vi "Count LEDs.vi"(8 "error in (no error)":errorcluster, 11 "LED Board Visual Test in":refnum<class "LED Board Test.lvclass">) -> (0 "error out":errorcluster, 2 "Fail Codes":string, 3 "Tests Passed":bool)   [LabVIEW 2015, in "LED Board Test.lvclass"]
uses:
  LED Board Test.lvclass
  LED Board Test.lvclass/LED Board Test.ctl
  Classes/Test Recipe/Class/Test Recipe.lvclass
  <vilib>/Cree, Inc/Cree Test Framework/Core Launcher/Core Launcher.lvlib
  <vilib>/Cree, Inc/Cree Test Framework/Classes/Data/Data Repo/Class/Data Repo.lvclass
  Classes/Application/Class/Application.lvclass
  Test Class/Test Class.lvclass
  Classes/Station Config/Class/Station Config.lvclass
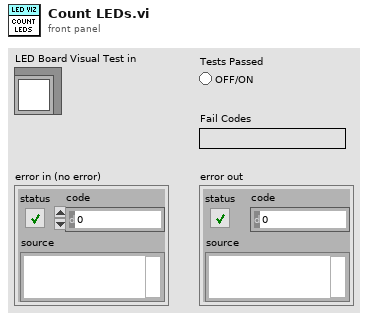
[diagram p1: front panel]
types:
  T1 = typedef "Application.lvlib/App Properties.lvclass/Class Properties -- Cluster.ctl" = cluster{"UUT Info":T2[], "Test Information":refnum<vi>, "Test Complete Event":refnum<user-event>, "Shop Floor System":refnum<class "Shop Floor System.lvclass">, "Gold Board":refnum<class "Golden Board.lvclass">, "Test Recipe":refnum<class "Test Recipe.lvclass">, "Instruments":refnum<class "Instrument.lvclass">[], "Mode":T3, "Test Results":T4[], "Station Config":refnum<class "Station Config.lvclass">}
  T2 = typedef "Application.lvlib/App Properties.lvclass/UUT Reference -- Cluster.ctl" = cluster{"Serial Number Reference":refnum<vi>, "Status Message Reference":refnum<vi>}
  T3 = typedef "Application.lvlib/Application.lvclass/Op Mode -- Enum.ctl" = u16
  T4 = typedef "Application.lvlib/App Properties.lvclass/Test Result -- Cluster.ctl" = cluster{"Position":i32, "Pass":bool, "Fail Codes":string}
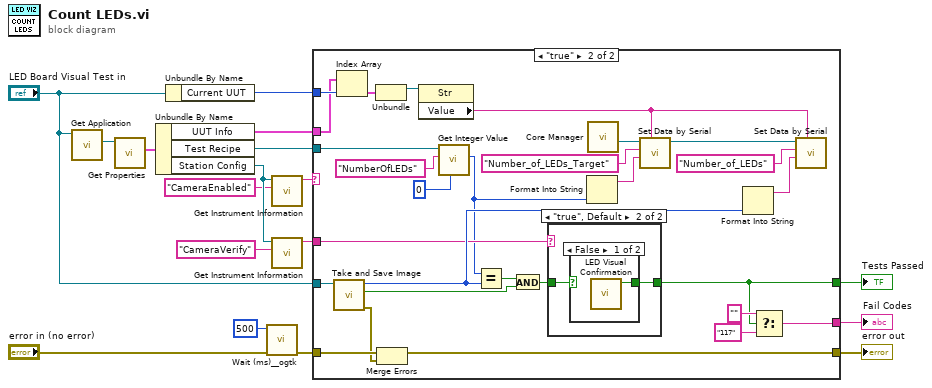
[diagram p0: block diagram]
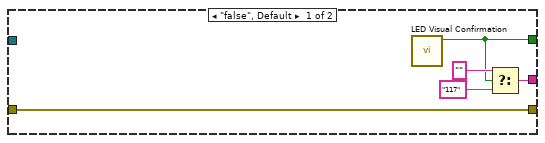
[diagram p2: hidden frame]
diagram:
  n1 = call "Get Application.vi"("Test Class in"="LED Board Visual Test in") -> ("Application.lvlib:Application.lvclass"=w3:refnum<class "Application.lvclass">)  [unwired: 9 in, 1 out]
  n2 = call "Get Properties.vi"("Acrobat Template in"=w3) -> ("Class Properties"=w2:T1)  [unwired: 8 in, 2 out]
  n3 = Unbundle By Name(w2) -> ("UUT Info"=w17:T2[], "Test Recipe"=w1:refnum<class "Test Recipe.lvclass">, "Station Config"=w15:refnum<class "Station Config.lvclass">)
  n4 = Unbundle By Name("LED Board Visual Test in") -> ("Current UUT"=w10:u32)
  n5 = call <userlib>:"Wait (ms)__ogtk.vi"("error in (no error)"="error in (no error)", "milliseconds to wait"=u32 500) -> ("error out"=w12:errorcluster)  [unwired: 8 in, 1 out]
  n6 = call "Get Instrument Information.vi"("Information Tag"="CameraEnabled", "Station Config in"=w15) -> ("Instrument Info"=w9:string)  [unwired: 8 in, 1 out]
  n7 = call "Get Instrument Information.vi"("Information Tag"="CameraVerify", "Station Config in"=w15) -> ("Instrument Info"=w16:string)  [unwired: 8 in, 1 out]
  n8 = case shown="\"true\"" w9 {
    tunnel: w1 -> [_ w48]
    tunnel: w12 -> [w22 w47]
    tunnel: [w22 w46] -> w5
    tunnel: [w19 w24] -> w6
    tunnel: [w18 w25] -> w7
    tunnel: "LED Board Visual Test in" -> [_ w40]
    tunnel: w10 -> [_ w35]
    tunnel: w16 -> [_ w36]
    tunnel: w17 -> [_ w34]
    frame "false", Default {
      n9 = call "LED Visual Confirmation.vi"() -> ("Pass"=w19:bool)  [unwired: 11 in]
      n10 = Select(t="" ("delimiter (Tab)"), s=w19, f="117" ("delimiter (Tab)")) -> (s? t:f=w18:string)
    }
    frame "true" {
      n11 = call "Take and Save Image.vi"("LED Board Visual Test in"=w40) -> ("error out"=w45:errorcluster, "Color Artifacts Found"=w23:bool, "LEDs Found"=w39:u32)  [unwired: 8 in]
      n12 = Index Array(array=w34, index=w35) -> (element=w33:T2)
      n13 = Unbundle(w33) -> ("Serial Number Reference"=w32:refnum<vi>)  [unwired: 1 out]
      n14 = Merge Errors(w47, w45) -> (w46:errorcluster)
      n15 = property class="Str"(reference=w32) -> ("Value"=w27:string)  [unwired: 1 in, 2 out]
      n16 = call "Get Integer Value.vi"("Default Value"=u32 0, "Name"="NumberOfLEDs", "Test Recipe in"=w48) -> ("Value"=w28:i32)  [unwired: 5 in, 3 out]
      n17 = Equal?(x=w28, y=w39) -> (x = y?=w38:bool)
      n18 = And(x=w38, y=w23) -> (x .and. y?=w37:bool)
      n19 = case shown="\"true\", Default" w36 {
        tunnel: [w51 w53] -> w24
        tunnel: w37 -> [w51 w52]
        frame "false" {
        }
        frame "true", Default {
          n20 = case shown="False" w52 {
            selector: w52 -> [_ w55]
            tunnel: [w54 w55] -> w53
            frame False {
              n21 = call "LED Visual Confirmation.vi"() -> ("Pass"=w54:bool)  [unwired: 11 in]
            }
            frame True {
            }
          }
        }
      }
      n22 = Format Into String(w28) -> (resulting string=w31:string)  [unwired: 3 in, 1 out]
      n23 = call <vilib>:"Core Manager.vi"() -> ("Data Repo"=w29:refnum<class "Data Repo.lvclass">)  [unwired: 7 in, 4 out]
      n24 = call <vilib>:"Set Data by Serial.vi"("Serial"=w27, "Value"=w31, "Header"="Number_of_LEDs_Target", "Acrobat Template in"=w29) -> ("Acrobat Template out"=w26:refnum<class "Data Repo.lvclass">)  [unwired: 6 in, 1 out]
      n25 = Format Into String(w39) -> (resulting string=w41:string)  [unwired: 3 in, 1 out]
      n26 = Select(t="" ("delimiter (Tab)"), s=w24, f="117" ("delimiter (Tab)")) -> (s? t:f=w25:string)
      n27 = call <vilib>:"Set Data by Serial.vi"("Serial"=w27, "Value"=w41, "Header"="Number_of_LEDs", "Acrobat Template in"=w26) -> ()  [unwired: 6 in, 2 out]
    }
  }
  "Fail Codes" <- w7
  "Tests Passed" <- w6
  "error out" <- w5
